vi "SCAN DONE.vi"(8 "error in (no error)":errorcluster, 9 "Boolean":bool, 10 "ScanQ in":refnum<queue>, 11 "Queue in":refnum<queue>) -> (0 "error out":errorcluster, 2 "ScanQ out":refnum<queue>, 3 "Queue out":refnum<queue>)   [LabVIEW 2025]
uses:
  STM-Auto-Project/QMH CTLS/Scan_Params (QMH).ctl
  LabVIEW VI's/Instrument VI's/Instrument Controls/Magnet Array.ctl
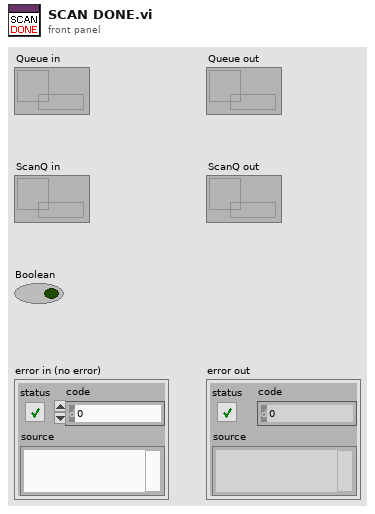
[diagram p1: front panel]
types:
  T1 = enum16{"SET FIELD", "SWEEP IDLE", "NEXT FIELD", "SWEEP DONE"}
  T2 = typedef "Magnet Array.ctl" = cluster{"Sweep States":enum16{"SET FIELD", "SWEEP IDLE", "NEXT FIELD", "SWEEP DONE"}, "VISA Connection":refnum<visa-resource-name>, "Fields(T)":dbl[]}
  T3 = enum16{"1. BIAS", "2. INIT_SCAN", "3. SCAN_IDLE", "4. INTER_SCAN", "5. NEW_COORDS_&_FRAME", "6. FINAL_SCAN", "7. STOP"}
  T4 = typedef "Scan_Params (QMH).ctl" = cluster{"Setpoint (I)":dbl[], "Bias (V)":dbl[], "Number of scans":u8, "Port number (3364)":u32, "Avoid zero threshold (V)":dbl, "Current State":enum16{"1. BIAS", "2. INIT_SCAN", "3. SCAN_IDLE", "4. INTER_SCAN", "5. NEW_COORDS_&_FRAME", "6. FINAL_SCAN", "7. POLL BIAS ", "8. STOP"}}
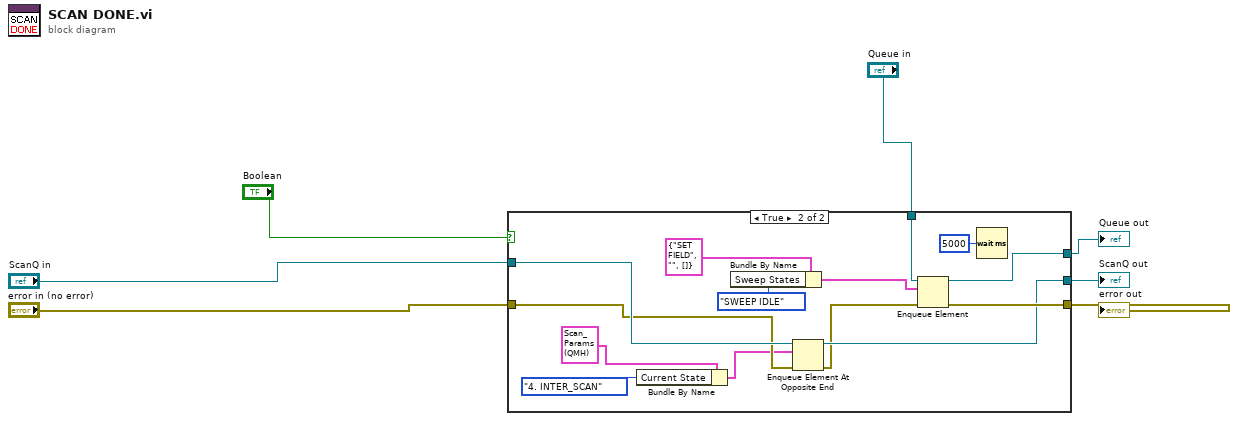
[diagram p0: block diagram]
diagram:
  n1 = case shown="True" "Boolean" {
    tunnel: [w9 w18] -> w4
    tunnel: "error in (no error)" -> [w8 w17]
    tunnel: "ScanQ in" -> [w9 w21]
    tunnel: [w8 w22] -> w5
    tunnel: "Queue in" -> [_ w13]
    tunnel: [_ w11] -> w7
    frame False {
    }
    frame True {
      n2 = Bundle By Name(cluster=T4 {"Setpoint (I)"=[], "Bias (V)"=[], "Number of scans"=1, "Port number (3364)"=3364, "Avoid zero threshold (V)"=0.004999999888241291, "Current State"=enum."1. BIAS"} ("element"), "Current State"=T3."4. INTER_SCAN") -> (w10:T4)
      n3 = Bundle By Name(cluster=T2 {"Sweep States"=enum."SET FIELD", "VISA Connection"="", "Fields(T)"=[]} ("element"), "Sweep States"=T1."SWEEP IDLE") -> (w14:T2)
      n4 = Enqueue Element At Opposite End(queue=w21, element=w10, error in (no error)=w17) -> (queue out=w18:refnum<queue>, error out=w16:errorcluster)  [unwired: 1 in, 1 out]
      n5 = Enqueue Element(queue=w13, element=w14, error in (no error)=w16) -> (queue out=w11:refnum<queue>, error out=w22:errorcluster)  [unwired: 1 in, 1 out]
      n6 = Wait (ms)(milliseconds to wait=u32 5000) -> ()  [unwired: 1 out]
    }
  }
  "Queue out" <- w7
  "error out" <- w5
  "ScanQ out" <- w4
